vi "Main.vi"() -> ()   [LabVIEW 2021]
uses:
  Controls/Runner's Data.ctl
  1/Control 2.ctl
  1/Control 5.ctl
  Controls/#type_def SM_States.ctl
  Controls/HR Data Structure.ctl
  Controls/Raw Data.ctl
panel:
  out "XY Graph":T1
  out "Heart Rate Zones":T2[][](array[typedef])
  out "Runners Data":T3
  out "BPM":cluster{"Time":timestamp[], "Bpm":i32[]}(graph)
  out "error out":errorcluster
  in  "error in":errorcluster
  in  "Stop Button":bool
  in  "Save Result":bool
  in  "New Training":bool
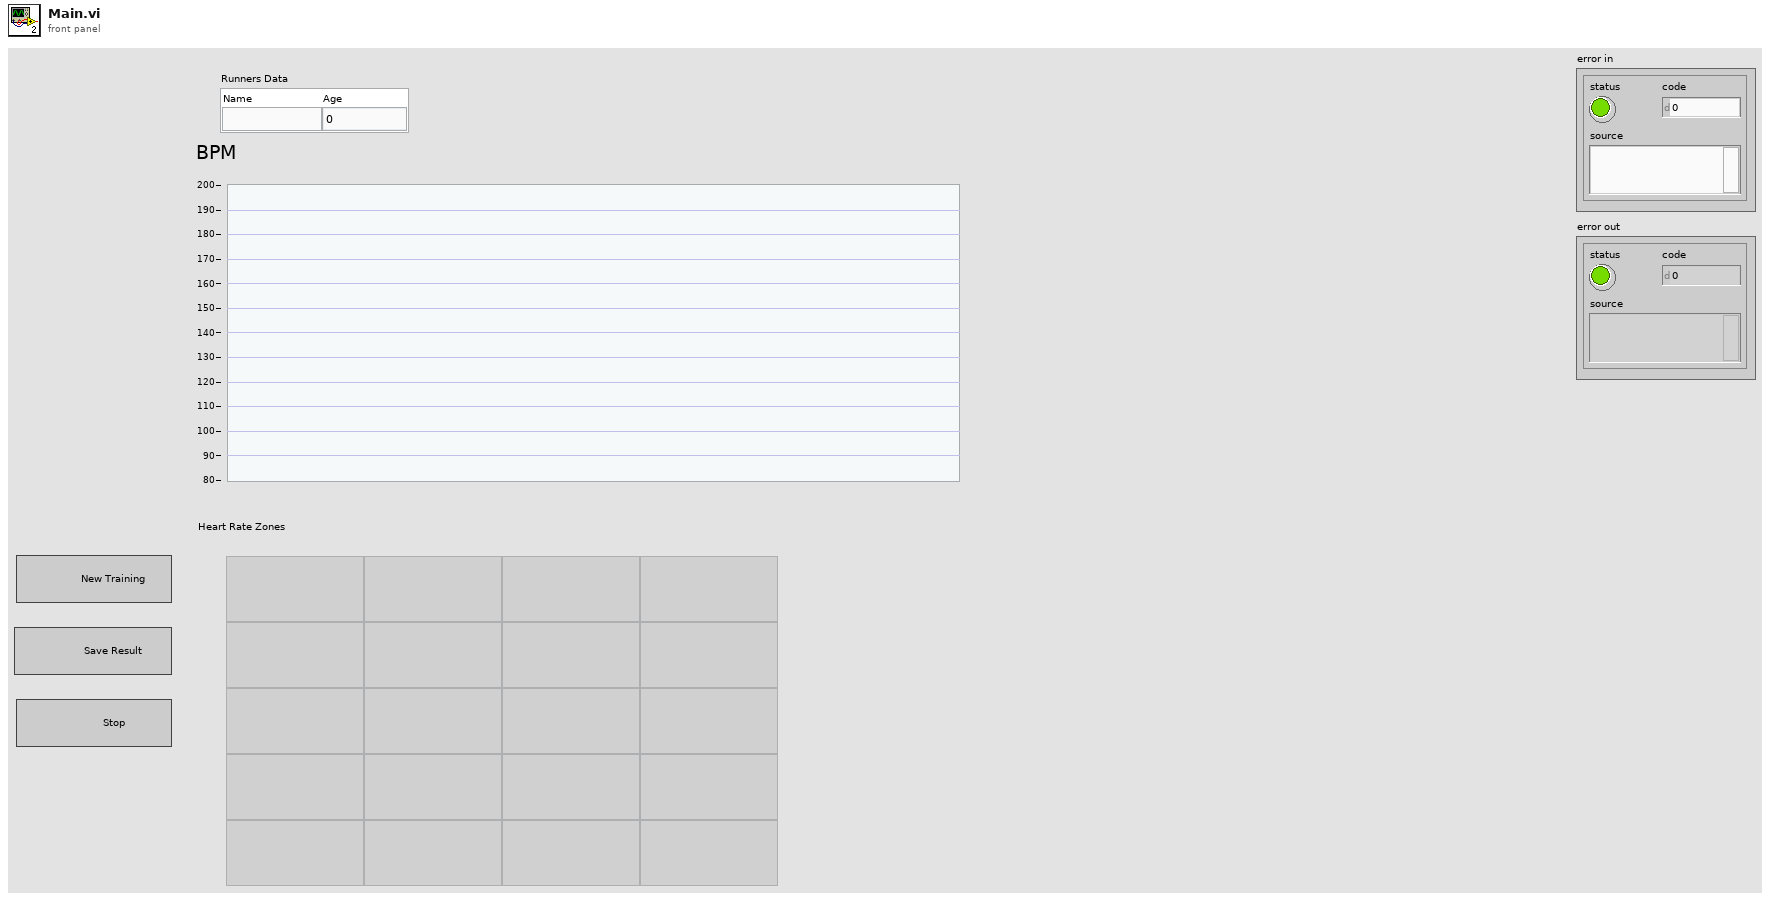
[diagram p1: front panel]
types:
  T1 = typedef "Control 5.ctl" = cluster{"Heart Rate Zone":i32[], " Total time in Zone (%) ":dbl[]}
  T2 = typedef "Control 2.ctl" = string
  T3 = typedef "Runner's Data.ctl" = cluster{"Name":string, "Age":i32}
  T4 = typedef "HR Data Structure.ctl" = cluster{"Runner's Data":T3, "HR Max":i32, "Raw Data":T5, "% HR MAX ":dbl[], "HR Zones Info":string[][], "Heart Rate Zones":dbl[]}
  T5 = typedef "Raw Data.ctl" = cluster{"Time":timestamp[], "Bpm":i32[]}
  T6 = typedef "#type_def SM_States.ctl" = enum16{"Application Error", "Init", "Idle", "Analyse New Training", "Save", "Error Handling", "Stop"}
  T7 = enum16{"open", "replace", "create", "open or create", "replace or create", "replace or create with confirmation"}
  T8 = cluster{"Heart Rate Zones No":dbl[], "Raw Data":T5, "HR Zones":string[][]}
  T9 = cluster{"reversed array":dbl[], "Heart Rate Zones No":dbl[]}
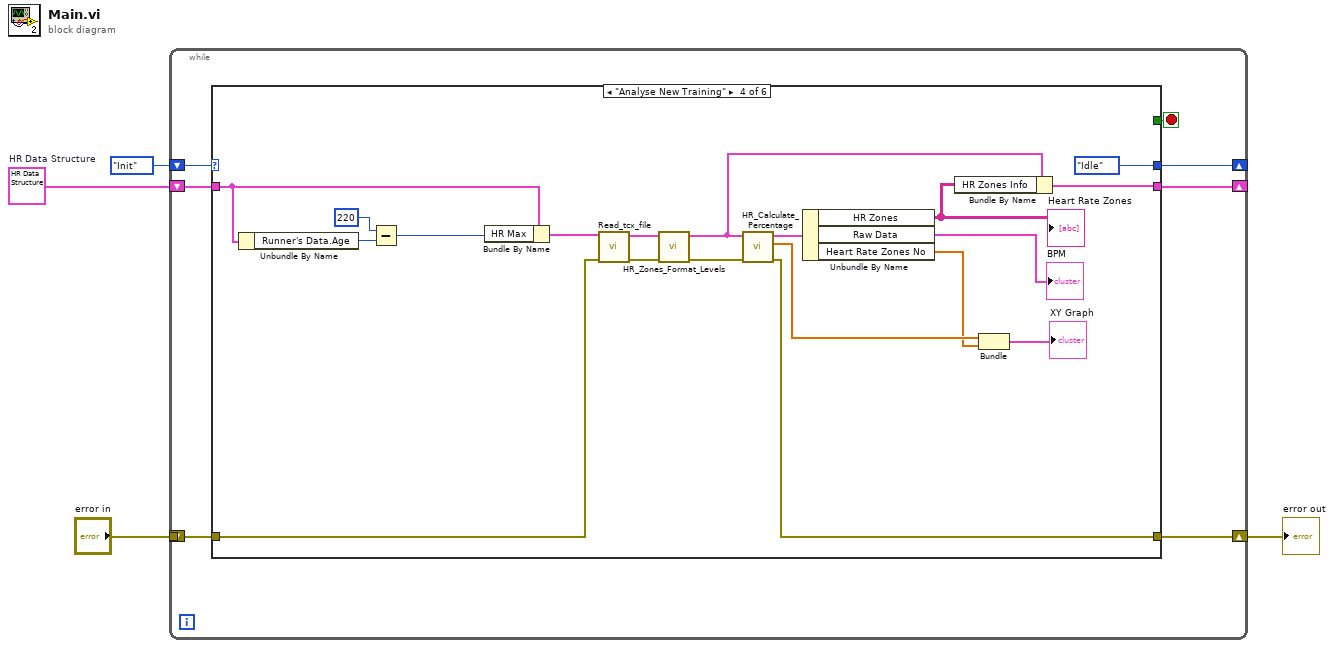
[diagram p0: block diagram]
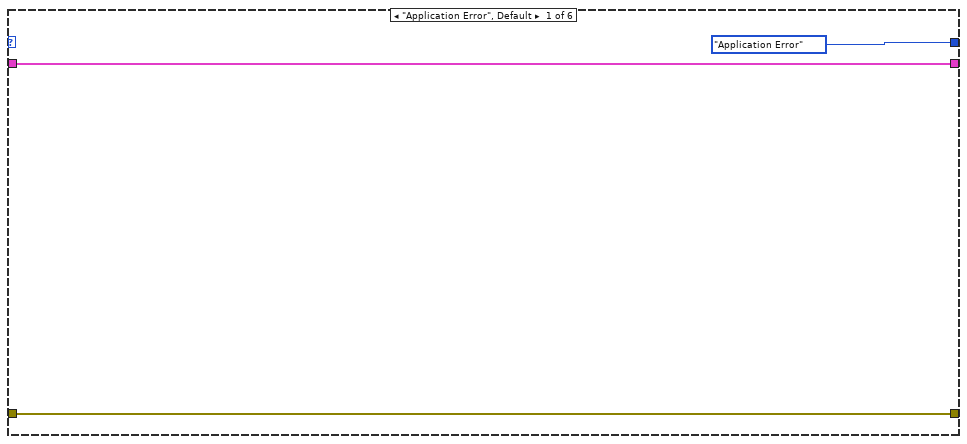
[diagram p2: hidden frame]
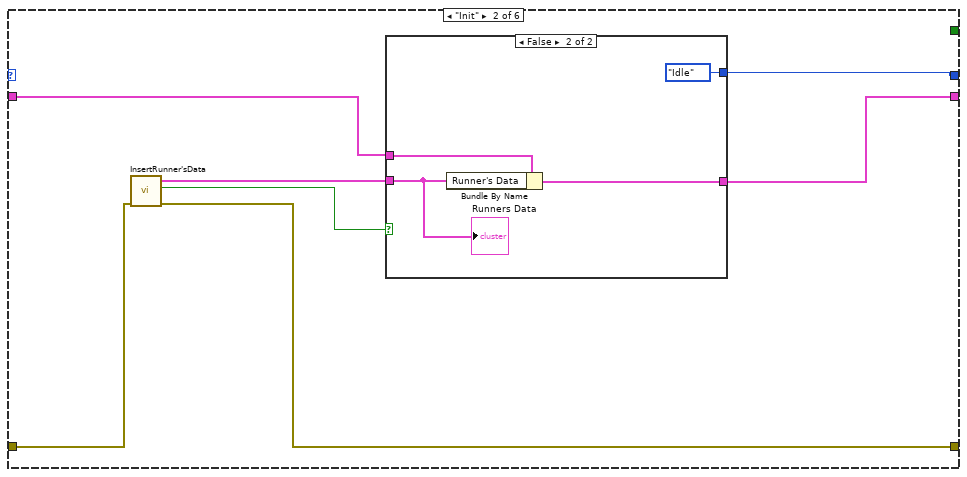
[diagram p3: hidden frame]
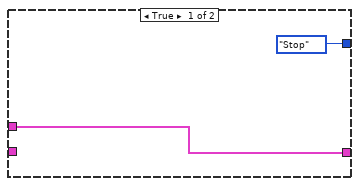
[diagram p4: hidden frame]
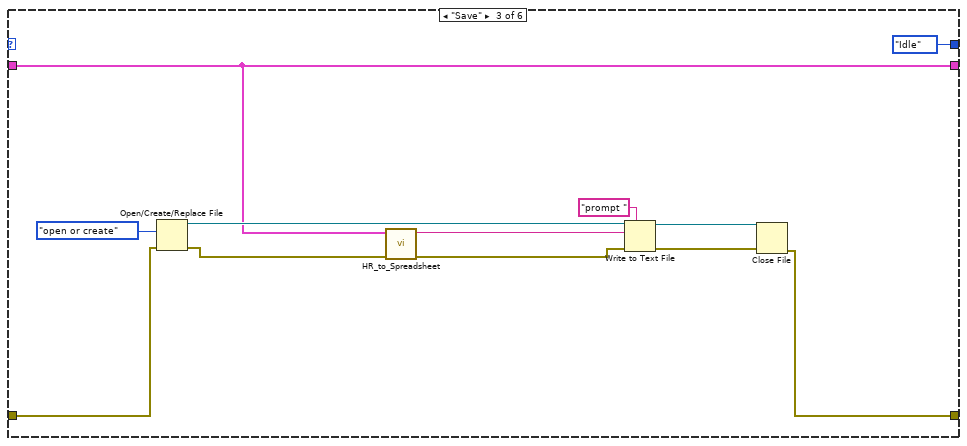
[diagram p5: hidden frame]
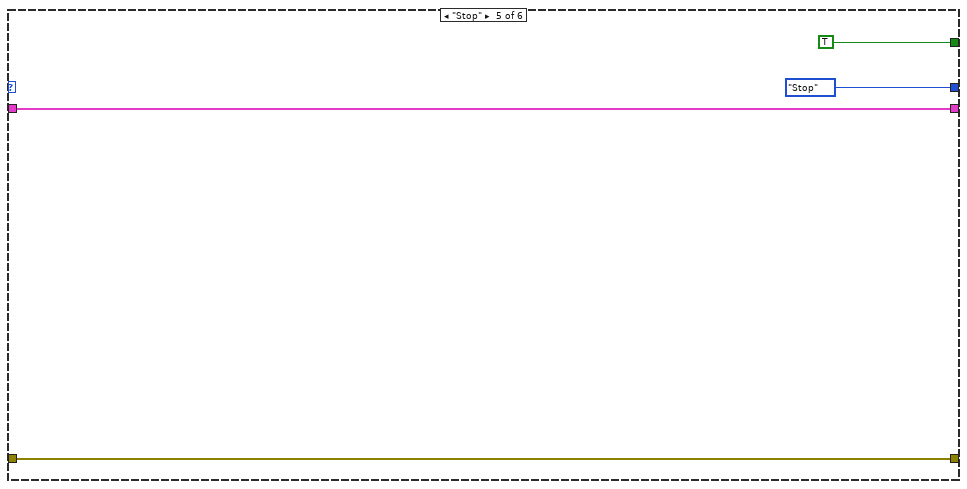
[diagram p6: hidden frame]
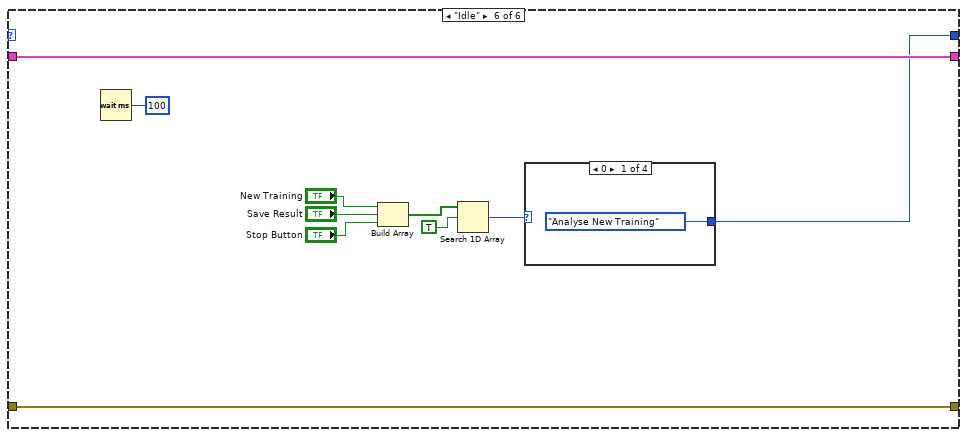
[diagram p7: hidden frame]
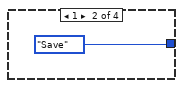
[diagram p8: hidden frame]
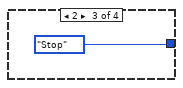
[diagram p9: hidden frame]
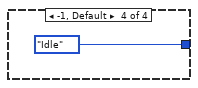
[diagram p10: hidden frame]
diagram:
  w1 = T4 data[18170B]  # HR Data Structure
  n1 = while {
    shift-right: [w10] -> _
    shift-left: #type_def_SM_States."Init" ("SM_States") -> [w11]
    shift-right: [w8] -> _
    shift-left: w1 -> [w7]
    tunnel: "error in" -> [w6]
    shift-right: [w5] -> w2
    shift-left: _ -> [_]
    stop <- w9 stop-if-true
    n2 = case shown="\"Analyse New Training\"" w11 {
      tunnel: [#type_def_SM_States."Application Error" ("SM_States") w15 #type_def_SM_States."Idle" ("SM_States") #type_def_SM_States."Idle" ("SM_States") #type_def_SM_States."Stop" ("SM_States") w64] -> w10
      tunnel: [_ _ _ _ TRUE _] -> w9
      tunnel: [w14 w20 w32 w40 w60 w72] -> w8
      tunnel: w7 -> [w14 w21 w32 w57 w60 w72]
      tunnel: [w13 w16 w34 w49 w59 w66] -> w5
      tunnel: w6 -> [w13 w17 w35 w52 w59 w66]
      frame "Application Error", Default {
      }
      frame "Init" {
        n3 = call "InsertRunner'sData.vi"("error in"=w17) -> ("error out"=w16:errorcluster, "Canceled?"=w18:bool, "Runners Data Out"=w19:T3)  [unwired: 8 in]
        n4 = case shown="False" w18 {
          tunnel: w21 -> [w23 w27]
          tunnel: [w23 w26] -> w20
          tunnel: w19 -> [_ w24]
          tunnel: [#type_def_SM_States."Stop" ("SM_States") #type_def_SM_States."Idle" ("SM_States")] -> w15
          frame True {
          }
          frame False {
            n5 = Bundle By Name(cluster=w27, "Runner's Data"=w24) -> (w26:T4)
            "Runners Data" <- w24
          }
        }
      }
      frame "Save" {
        n6 = Open/Create/Replace File(error in=w35, operation (0:open)=T7."open or create") -> (refnum out=w37:refnum<file>, error out=w29:errorcluster)  [unwired: 4 in, 1 out]
        n7 = call "HR_to_Spreadsheet.vi"("error in (no error)"=w29, "HR Data Structure"=w32) -> ("error out"=w28:errorcluster, "HR Zones Info SpreadSheet"=w31:string)  [unwired: 8 in]
        n8 = Write to Text File(prompt (Choose or enter file path)="prompt ", file (use dialog)=w37, text=w31, error in=w28) -> (refnum out=w36:refnum<file>, error out=w30:errorcluster)  [unwired: 1 out]
        n9 = Close File(refnum=w36, error in=w30) -> (error out=w34:errorcluster)  [unwired: 1 out]
      }
      frame "Analyse New Training" {
        n10 = Unbundle By Name(w57) -> ("Runner's Data.Age"=w56:i32)
        n11 = Subtract(x=220, y=w56) -> (x-y=w43:i32)
        n12 = Bundle By Name(cluster=w57, "HR Max"=w43) -> (w54:T4)
        n13 = call "Read_tcx_file.vi"("error in (no error)"=w52, "HR Data Structure"=w54) -> ("error out"=w51:errorcluster, "HR Data Structure 2"=w53:T4)  [unwired: 8 in]
        n14 = call "HR_Zones_Format_Levels.vi"("error in (no error)"=w51, "HR Data Structure"=w53) -> ("error out"=w50:errorcluster, "HR Data Structure 2"=w42:T4)  [unwired: 8 in]
        n15 = call "HR_Calculate_Percentage.vi"("error in (no error)"=w50, "HR Data Structure in"=w42) -> ("error out"=w49:errorcluster, "reversed array"=w46:dbl[], "ShowCluster"=w48:T8)  [unwired: 6 in]
        n16 = Unbundle By Name(w48) -> ("HR Zones"=w41:string[][], "Raw Data"=→"BPM":T5, "Heart Rate Zones No"=w45:dbl[])
        "Heart Rate Zones" <- w41
        n17 = Bundle By Name(cluster=w42, "HR Zones Info"=w41) -> (w40:T4)
        n18 = Bundle("reversed array"=w46, "Heart Rate Zones No"=w45) -> (→"XY Graph":T9)  [unwired: 1 in]
      }
      frame "Stop" {
      }
      frame "Idle" {
        n19 = Wait (ms)(milliseconds to wait=u32 100) -> ()  [unwired: 1 out]
        n20 = Build Array("New Training", "Save Result", "Stop Button") -> (w68:bool[])
        n21 = Search 1D Array(1D array=w68, element=TRUE) -> (index of element=w65:i32)  [unwired: 1 in]
        n22 = case shown="0" w65 {
          tunnel: [#type_def_SM_States."Analyse New Training" ("SM_States") #type_def_SM_States."Save" ("SM_States") #type_def_SM_States."Stop" ("SM_States") #type_def_SM_States."Idle" ("SM_States")] -> w64
          frame 0 {
          }
          frame 1 {
          }
          frame 2 {
          }
          frame -1, Default {
          }
        }
      }
    }
  }
  "error out" <- w2
